vi "Swerve Math.vi"(9 "Yaw":dbl=-5.71) -> (3 "Swerve Math Ouput":dbl[](array[numeric])=[0.0, 0.0, 0.0, 0.0, 0.0, 10.75, 16.677080080157918, 12.75])   [LabVIEW 2018]
uses:
  Drive Train Global.vi
  Robot Information/Robot Information Global.vi
  <vilib>/addons/control/pid/pid.llb/PID (DBL).vi
  <vilib>/addons/control/pid/NI_PID_pid.lvlib
panel:
  in  "PID gains":T1={"proportional gain (Kc)"=0.03, "integral time (Ti, min)"=0.0, "derivative time (Td, min)"=0.001} {"derivative time (Td, min)" format="%.3f"; "integral time (Ti, min)" format="%.3f"; "proportional gain (Kc)" format="%.3f"}
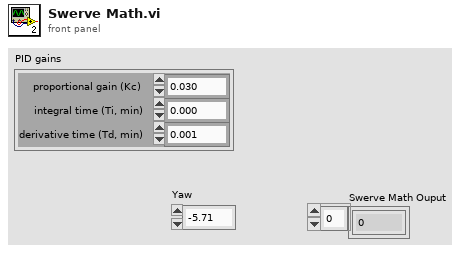
[diagram p1: front panel]
types:
  T1 = cluster{"proportional gain (Kc)":dbl, "integral time (Ti, min)":dbl, "derivative time (Td, min)":dbl}
  T2 = cluster{"Rollover":dbl, "Yaw":dbl, "Cont Yaw":dbl}
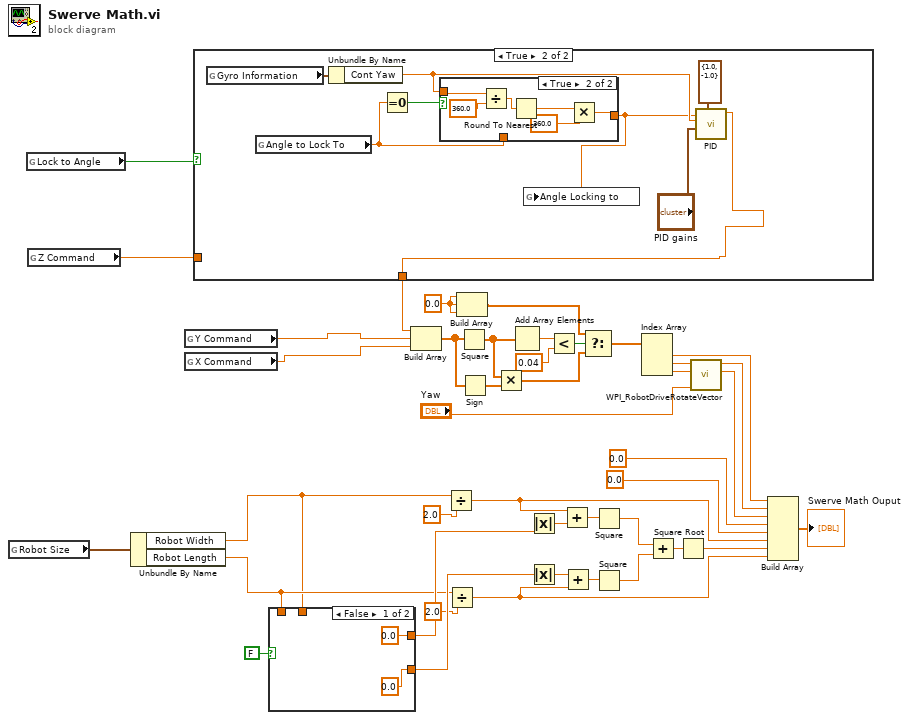
[diagram p0: block diagram]
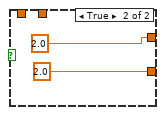
[diagram p2: hidden frame]
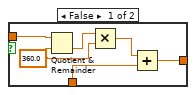
[diagram p4: hidden frame]
diagram:
  w17 = 0.0 ("element")
  n1 = global read "Robot Information Global.vi" "Robot Size"() -> (w22:cluster{"Robot Width":dbl, "Robot Length":dbl})
  n2 = global read "Drive Train Global.vi" "Lock to Angle"() -> (w9:bool)
  n3 = global read "Drive Train Global.vi" "Z Command"() -> (w10:dbl)
  n4 = Unbundle By Name(w22) -> ("Robot Width"=w2:dbl, "Robot Length"=w5:dbl)
  n5 = global read "Drive Train Global.vi" "Y Command"() -> (w7:dbl)
  n6 = global read "Drive Train Global.vi" "X Command"() -> (w6:dbl)
  n7 = case shown="True" w9 {
    tunnel: [w43 w44] -> w8
    tunnel: w10 -> [w43 _]
    frame False {
    }
    frame True {
      n8 = global read "Drive Train Global.vi" "Gyro Information"() -> (w51:T2)
      n9 = global read "Drive Train Global.vi" "Angle to Lock To"() -> (w46:dbl)
      n10 = Unbundle By Name(w51) -> ("Cont Yaw"=w48:dbl)
      n11 = Equal To 0?(x=w46) -> (x = 0?=w45:bool)
      n12 = case shown="True" w45 {
        tunnel: w48 -> [w57 w63]
        tunnel: w46 -> [w56 _]
        tunnel: [w55 w58] -> w47
        frame False {
          w53 = 360.0 ("y")
          n13 = Quotient & Remainder(x=w57, y=w53) -> (floor(x/y)=w54:dbl)  [unwired: 1 out]
          n14 = Multiply(x=w54, y=w53) -> (x*y=w52:dbl)
          n15 = Add(x=w52, y=w56) -> (x+y=w55:dbl)
        }
        frame True {
          n16 = Divide(x=w63, y=360.0) -> (x/y=w61:dbl)
          n17 = Round To Nearest(number=w61) -> (nearest integer value=w60:dbl)
          n18 = Multiply(x=w60, y=360.0) -> (x*y=w58:dbl)
        }
      }
      n19 = global write "Drive Train Global.vi" "Angle Locking to"(w47) -> ()
      n20 = call-poly <vilib>:"PID.vi"("output range"=cluster{"output high":dbl, "output low":dbl} {"output high"=1.0, "output low"=-1.0}, "PID gains"="PID gains", "process variable"=w48, "setpoint"=w47) -> ("output"=w44:dbl)  [unwired: 6 in, 1 out]
    }
  }
  n21 = case shown="False" FALSE {
    tunnel: [0.0 ("Rot. Point X") 2.0 ("y")] -> w35
    tunnel: [0.0 ("Rot. Point Y") 2.0 ("y")] -> w34
    tunnel: w5 -> [_ _]
    tunnel: w2 -> [_ _]
    frame False {
    }
    frame True {
    }
  }
  n22 = Build Array(w8, w7, w6) -> (w13:dbl[])
  n23 = Divide(x=w2, y=2.0) -> (x/y=w30:dbl)
  n24 = Divide(x=w5, y=2.0) -> (x/y=w28:dbl)
  n25 = Build Array(w17, w17, w17) -> (w18:dbl[])
  n26 = Square(x=w13) -> (x^2=w15:dbl[])
  n27 = Sign(1:w13) -> (0:w16:dbl[])
  n28 = Multiply(x=w15, y=w16) -> (x*y=w14:dbl[])
  n29 = Add Array Elements(numeric array=w15) -> (sum=w21:dbl)
  n30 = Absolute Value(x=w35) -> (abs(x)=w42:dbl)
  n31 = Absolute Value(x=w34) -> (abs(x)=w40:dbl)
  n32 = Less?(x=w21, y=0.04 ("x")) -> (x < y?=w19:bool)
  n33 = Add(x=w30, y=w42) -> (x+y=w41:dbl)
  n34 = Add(x=w40, y=w28) -> (x+y=w39:dbl)
  n35 = Select(t=w18, s=w19, f=w14) -> (s? t:f=w26:dbl[])
  n36 = Square(x=w41) -> (x^2=w37:dbl)
  n37 = Square(x=w39) -> (x^2=w38:dbl)
  n38 = Index Array(array=w26) -> (element #1=w24:dbl, element #2=w27:dbl, element #3=w31:dbl)  [unwired: 3 in]
  n39 = Add(x=w37, y=w38) -> (x+y=w36:dbl)
  n40 = Square Root(x=w36) -> (sqrt(x)=w29:dbl)
  n41 = call <vilib>:"WPI_RobotDriveRotateVector.vi"("Angle"="Yaw", "X"=w31, "Y"=w27) -> ("X'"=w25:dbl, "Y'"=w23:dbl)  [unwired: 7 out]
  n42 = Build Array(w24, w23, w25, 0.0 ("element"), 0.0 ("element"), w30, w29, w28) -> (→"Swerve Math Ouput":dbl[])
